vi "Color Tree Items.vi"(8 "error in (no error)":errorcluster, 10 "Tree Map":map{path, T1}(c390), 11 "Tree Refnum":refnum<vi>) -> (0 "error out":errorcluster, 3 "Tree Refnum out":refnum<vi>)   [LabVIEW 2023]
doc: "Colors the tree items based on several criteria."
uses:
  CTLs/Tree Map Value.ctl
  <userlib>/_OpenG.lib/file/file.llb/Strip Path Extension - Path__ogtk.vi
  <userlib>/_OpenG.lib/array/array.llb/Filter 1D Array with Scalar (I32)__ogtk.vi
  <userlib>/_OpenG.lib/array/array.llb/Index 1D Array Elements (Path)__ogtk.vi
  <userlib>/_OpenG.lib/array/array.llb/Filter 1D Array with Scalar (Path)__ogtk.vi
  <userlib>/_OpenG.lib/file/file.llb/Strip Path - Arrays__ogtk.vi
  <userlib>/_OpenG.lib/array/array.llb/openg_array.lvlib
  <userlib>/_OpenG.lib/file/file.llb/openg_file.lvlib
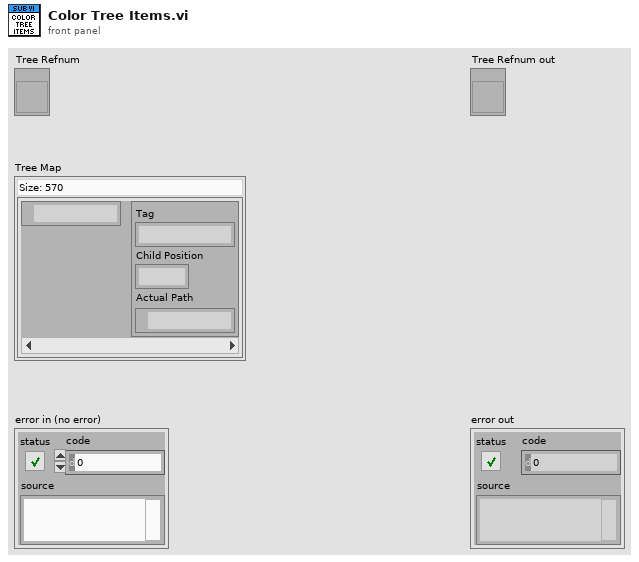
[diagram p1: front panel]
types:
  T1 = typedef "Tree Map Value.ctl" = cluster{"Tag":string, "Child Position":i32, "Actual Path":path}
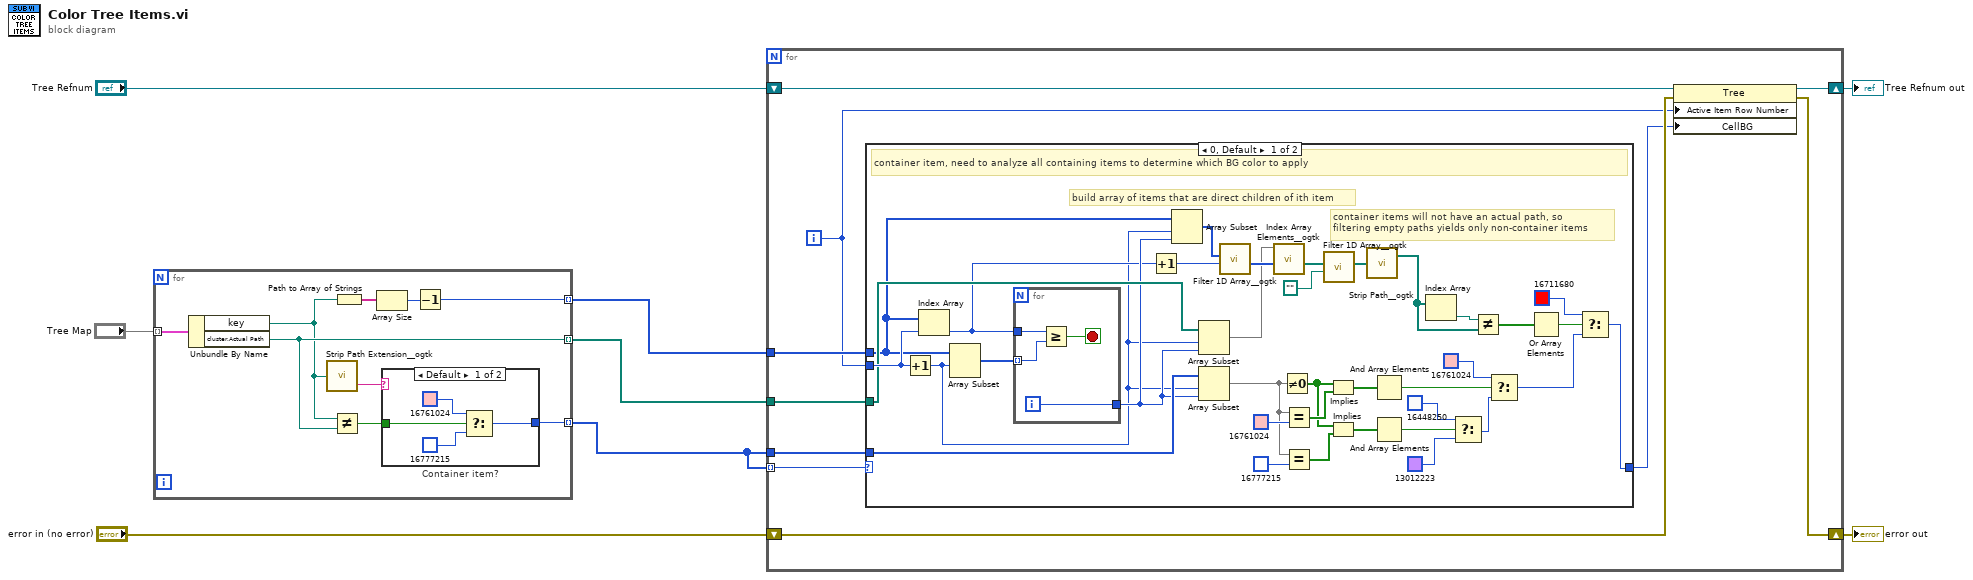
[diagram p0: block diagram]
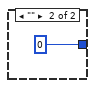
[diagram p2: hidden frame]
diagram:
  n1 = for {
    tunnel: "Tree Map" -> [w17] mode=indexing
    tunnel: [w14] -> w5 mode=indexing
    tunnel: [w13] -> w6 mode=indexing
    tunnel: [w9] -> w7 mode=indexing
    n2 = Unbundle By Name(w17) -> ("key"=w12:path, "cluster.Actual Path"=w13:path)
    n3 = call-poly <userlib>:"Strip Path Extension__ogtk.vi"("path"=w12) -> ("extension"=w10:string)  [unwired: 1 out]
    n4 = Not Equal?(x=w12, y=w13) -> (x != y?=w11:bool)
    n5 = Path to Array of Strings(0:w12) -> (2:w16:string[])  [unwired: 1 out]
    n6 = Array Size(array=w16) -> (size(s)=w15:i32)
    n7 = case "Container item?" shown="Default" w10 {
      tunnel: [w21 u32 0] -> w9
      tunnel: w11 -> [w18 _]
      frame Default {
        n8 = Select(t=u32 16761024, s=w18, f=u32 16777215) -> (s? t:f=w21:u32)
      }
      frame "" {
      }
    }
    n9 = Decrement(x=w15) -> (x-1=w14:i32)
  }
  n10 = for {
    tunnel: w7 -> [w29] mode=indexing
    tunnel: w5 -> [w28]
    tunnel: w7 -> [w25]
    tunnel: w6 -> [w24]
    shift-right: [w32] -> w3
    shift-left: "error in (no error)" -> [w31]
    shift-right: [w23] -> w2
    shift-left: "Tree Refnum" -> [w30]
    i -> [w27]
    n11 = case shown="0, Default" w29 {
      selector: w29 -> [_ w73]
      tunnel: w28 -> [w40 _]
      tunnel: w27 -> [w68 _]
      tunnel: [w48 w73] -> w26
      tunnel: w25 -> [w67 _]
      tunnel: w24 -> [w51 _]
      frame 0, Default {
        # "container items will not have an actual path, so\nfiltering empty paths yields only non-container items"
        # "build array of items that are direct children of ith item"
        # "container item, need to analyze all containing items to determine which BG color to apply"
        n12 = Increment(x=w68) -> (x+1=w39:i32)
        n13 = Index Array(array=w40, index=w68) -> (element=w42:i32)
        n14 = Array Subset(array=w40, index=w39) -> (w45:i32[])  [unwired: 1 in]
        n15 = for {
          tunnel: w45 -> [w69] mode=indexing
          tunnel: w42 -> [w72]
          tunnel: [w70] -> w44
          i -> [w70]
          stop <- w71 stop-if-true
          n16 = Greater Or Equal?(x=w72, y=w69) -> (x >= y?=w71:bool)
        }
        n17 = Increment(x=w42) -> (x+1=w41:i32)
        n18 = Array Subset(array=w40, index=w39, length=w44) -> (w43:i32[])
        n19 = Array Subset(array=w51, index=w39, length=w44) -> (w37:path[])
        n20 = Array Subset(array=w67, index=w39, length=w44) -> (w62:u32[])
        n21 = call-poly <userlib>:"Filter 1D Array__ogtk.vi"("items to filter"=w41, "array"=w43) -> ("filtered item indices"=w38:i32[])  [unwired: 4 in, 1 out]
        n22 = call-poly <userlib>:"Index Array Elements__ogtk.vi"("indices"=w38, "array"=w37) -> ("elements"=w36:path[])  [unwired: 9 in]
        n23 = Not Equal To 0?(x=w62) -> (x != 0?=w50:bool[])
        n24 = Equal?(x=w62, y=u32 16761024) -> (x = y?=w65:bool[])
        n25 = Equal?(x=w62, y=u32 16777215) -> (x = y?=w63:bool[])
        n26 = call-poly <userlib>:"Filter 1D Array__ogtk.vi"("items to filter"=path "", "array"=w36) -> ("filtered array"=w34:path[])  [unwired: 4 in, 1 out]
        n27 = Implies(1:w65, 2:w50) -> (0:w61:bool[])
        n28 = Implies(1:w63, 2:w50) -> (0:w60:bool[])
        n29 = call-poly <userlib>:"Strip Path__ogtk.vi"("path"=w34) -> ("stripped path"=w33:path[])  [unwired: 1 out]
        n30 = And Array Elements(Boolean array=w61) -> (logical AND=w59:bool)
        n31 = And Array Elements(Boolean array=w60) -> (logical AND=w56:bool)
        n32 = Index Array(array=w33) -> (element=w47:path)  [unwired: 1 in]
        n33 = Select(t=u32 16448250, s=w56, f=u32 13012223) -> (s? t:f=w55:u32)
        n34 = Not Equal?(x=w47, y=w33) -> (x != y?=w46:bool[])
        n35 = Select(t=u32 16761024, s=w59, f=w55) -> (s? t:f=w52:u32)
        n36 = Or Array Elements(Boolean array=w46) -> (logical OR=w49:bool)
        n37 = Select(t=u32 16711680, s=w49, f=w52) -> (s? t:f=w48:u32)
      }
      frame 1.. {
        # "not a container item, apply BG color determined in previous loop"
      }
    }
    n38 = property class="Tree"(reference=w30, error in=w31, "Active Item Row Number"=w27, "CellBG"=w26) -> (reference out=w23:refnum<vi>, error out=w32:errorcluster)
  }
  "error out" <- w3
  "Tree Refnum out" <- w2
